vi "Change Paths Directory.vi"(9 "VI Refnum":refnum<vi>, 10 "config path":path, 11 "Bordeaux paths directory":path) -> (3 "Bordeaux paths out":path)   [LabVIEW 2025]
uses:
  <vilib>/Utility/sysdir.llb/System Directory Type.ctl
  <vilib>/Utility/config.llb/Write Key (Path).vi
  <vilib>/Utility/config.llb/Read Key (Path).vi
  <vilib>/Utility/config.llb/NI_LVConfig.lvlib
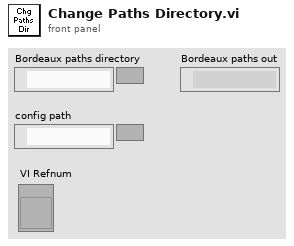
[diagram p1: front panel]
types:
  T1 = typedef "System Directory Type.ctl" = i32
  T2 = typedef "NI_LVConfig.lvlib/Config Data RefNum.ctl" = refnum<k1>
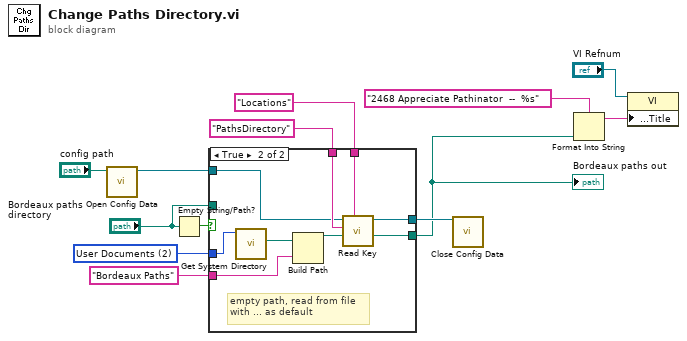
[diagram p0: block diagram]
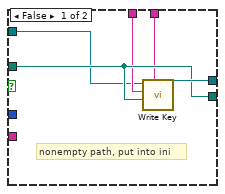
[diagram p2: hidden frame]
diagram:
  w8 = T1 2 items=["User Home"=0, "User Desktop"=1, "User Documents"=2, "User Application Data"=3, "User Preferences"=4, "User Temporary"=5, "Public Documents"=6, "Public Application Data"=7, "Public Preferences"=8, "Public Cache"=13, "System Core Libraries"=9, "System Installed Libraries"=10, "Application Files"=11, "Boot Volume Root"=12] ("system directory type")
  n1 = call <vilib>:"Open Config Data.vi"("configuration file path"="config path") -> ("refnum"=w3:T2)  [unwired: 8 in, 2 out]
  n2 = Empty String/Path?(string/path="Bordeaux paths directory") -> (empty?=w10:bool)
  n3 = case shown="True" w10 {
    tunnel: "Bordeaux Paths" ("format string") -> [_ w26]
    tunnel: w8 -> [_ w25]
    tunnel: [w17 w23] -> w2
    tunnel: [w18 w22] -> w7
    tunnel: "Bordeaux paths directory" -> [w17 _]
    tunnel: "Locations" ("section") -> [w16 w21]
    tunnel: "PathsDirectory" ("key") -> [w15 w20]
    tunnel: w3 -> [w14 w19]
    frame False {
      # "nonempty path, put into ini"
      n4 = call-poly <vilib>:"Write Key.vi"("section"=w16, "value"=w17, "key"=w15, "refnum"=w14) -> ("refnum out"=w18:T2)  [unwired: 5 in, 2 out]
    }
    frame True {
      # "empty path, read from file\nwith ... as default"
      n5 = call <vilib>:"Get System Directory.vi"("system directory type"=w25) -> ("system directory"=w27:path)  [unwired: 10 in]
      n6 = Build Path(base path=w27, name or relative path=w26) -> (appended path=w24:path)
      n7 = call-poly <vilib>:"Read Key.vi"("section"=w21, "default value"=w24, "key"=w20, "refnum"=w19) -> ("value"=w23:path, "refnum out"=w22:T2)  [unwired: 4 in, 2 out]
    }
  }
  "Bordeaux paths out" <- w2
  n8 = call <vilib>:"Close Config Data.vi"("refnum"=w7) -> ()  [unwired: 9 in, 2 out]
  n9 = Format Into String(format string="2468 Appreciate Pathinator  --  %s", w2) -> (resulting string=w11:string)  [unwired: 2 in, 1 out]
  n10 = property class="VI"(reference="VI Refnum", "Front Panel.Title"=w11) -> ()  [unwired: 1 in, 2 out]
